vi "DrawCross.vi"(6 "color(black)":u32(colorbox)=13816530, 8 "Width":u32, 9 "Height":u32, 10 "new position":cluster{"x":i16, "y":i16}, 11 "picture":picture) -> (3 "new picture":picture)   [LabVIEW 2023]
doc: "Draws a cross to x and y axis."
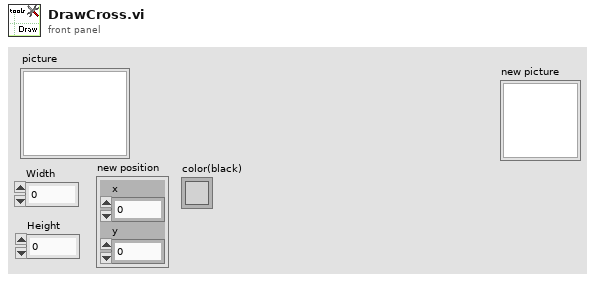
[diagram p1: front panel]
types:
  T1 = cluster{"Width":u16, "Style":enum32{"Solid", "Dash", "Dot", "DashDot", "DashDotDot"}}
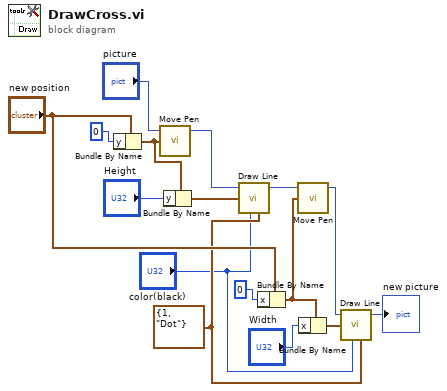
[diagram p0: block diagram]
diagram:
  w2 = T1 {"Width"=1, "Style"=enum."Dot"} ("pen")
  n1 = Bundle By Name(cluster="new position", "y"=i16 0) -> (w6:cluster{"x":i16, "y":i16})
  n2 = call <vilib>:"Move Pen.vi"("new position"=w6, "picture"="picture") -> ("new picture"=w4:picture)  [unwired: 3 in]
  n3 = Bundle By Name(cluster=w6, "y"="Height") -> (w9:cluster{"x":i16, "y":i16})
  n4 = call <vilib>:"Draw Line.vi"("picture"=w4, "end point"=w9, "color(black)"="color(black)", "pen"=w2) -> ("new picture"=w15:picture)  [unwired: 5 in]
  n5 = Bundle By Name(cluster="new position", "x"=i16 0 ("y")) -> (w12:cluster{"x":i16, "y":i16})
  n6 = call <vilib>:"Move Pen.vi"("new position"=w12, "picture"=w15) -> ("new picture"=w8:picture)  [unwired: 3 in]
  n7 = Bundle By Name(cluster=w12, "x"="Width") -> (w13:cluster{"x":i16, "y":i16})
  n8 = call <vilib>:"Draw Line.vi"("picture"=w8, "end point"=w13, "color(black)"="color(black)", "pen"=w2) -> ("new picture"=→"new picture":picture)  [unwired: 5 in]
